vi "GetScanParametersFromIntesityGraph.vi"(10 "FromCenter":bool=TRUE, 11 "IntensityGraph":refnum<vi>) -> (0 "Height":sgl, 1 "Width":sgl, 2 "Y":sgl, 3 "X":sgl)   [LabVIEW 2017]
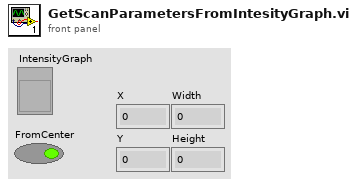
[diagram p1: front panel]
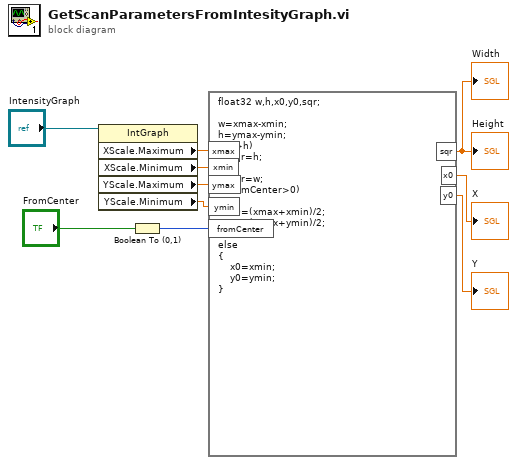
[diagram p0: block diagram]
diagram:
  n1 = property on="Property Node" class="IntGraph"(reference="IntensityGraph") -> ("XScale.Maximum"=w6:dbl, "XScale.Minimum"=w7:dbl, "YScale.Maximum"=w8:dbl, "YScale.Minimum"=w9:dbl)  [unwired: 1 in, 2 out]
  n2 = Boolean To (0,1)(Boolean="FromCenter") -> (0, 1=w3:i16)
  n3 = formula code="float32 w,h,x0,y0,sqr;\n\nw=xmax-xmin;\nh=ymax-ymin;\nif(w>h)\n    sqr=h;\nelse\n    sqr=w;\nif(fromCenter>0)\n{\n    x0=(xmax+xmin)/2;\n    y0=(ymax+ymin)/2;\n}\nelse\n{\n    x0=xmin;\n    y0=ymin;\n}"("xmax"=w6, "xmin"=w7, "ymax"=w8, "ymin"=w9, "fromCenter"=w3) -> ("sqr"=→"Width" →"Height":sgl, "x0"=→"X":sgl, "y0"=→"Y":sgl)
